vi "main OP300.vi"() -> ()   [LabVIEW 2020]
uses:
  SubVI/OP300ZP_state.ctl
  <vilib>/Sylvain.lib/02 SLIM ZEN WS 500/SubVi/FGV.ctl
  <vilib>/Sylvain.lib/02 SLIM ZEN WS 500/SubVi/VG_progressBar.vi
  SubVI/CheminDeBase.vi
  VG/PN.vi
  VG/IS30%.vi
  VG/R.vi
panel:
  out "IS30% ?":bool
  out "Cluster":T1
  out "VISA OUT":T2
  out "progression":u8(slide) scale=0.0..100.0
  out "PN":string
  out "errout 2":errorcluster={"status"=TRUE, "code"=0, "source"="PCAN_CHANNEL ILLEGAL"} caption="errout"
  out "errout":errorcluster caption="sortie d'erreur"
  out "STOP":bool
  out "TOP":string
  out "DRAW":picture
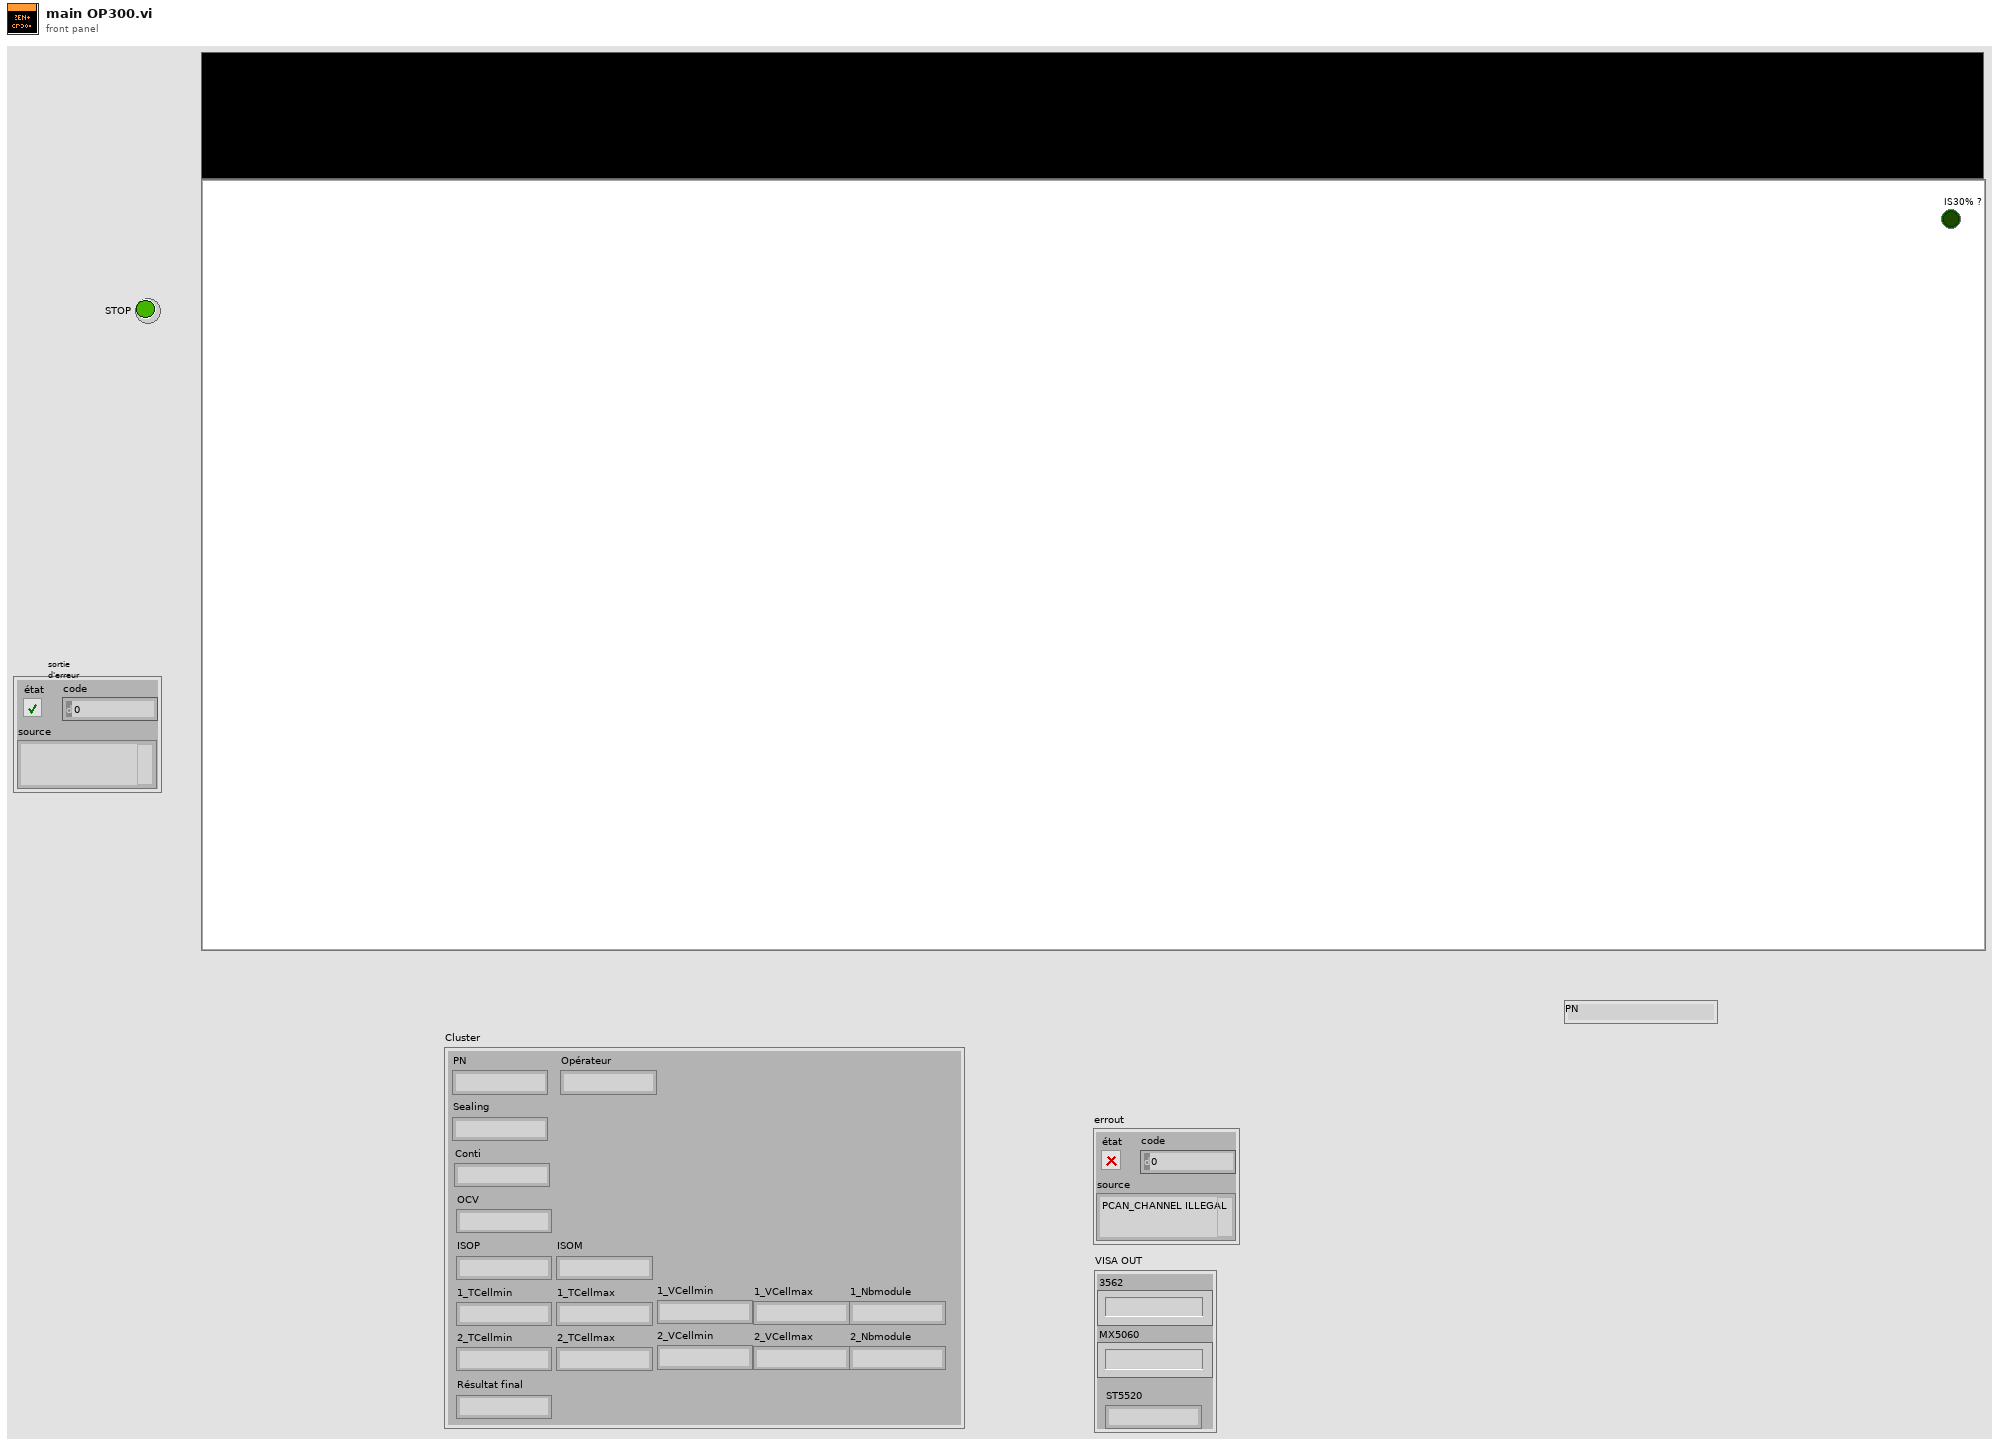
[diagram p1: front panel]
types:
  T1 = cluster{"PN":string, "Opérateur":string, "Sealing":string, "Conti":string, "OCV":string, "ISOP":string, "ISOM":string, "1_TCellmin":string, "1_TCellmax":string, "1_VCellmin":string, "1_VCellmax":string, "1_Nbmodule":string, "2_TCellmin":string, "2_TCellmax":string, "2_VCellmin":string, "2_VCellmax":string, "2_Nbmodule":string, "Résultat final":string}
  T2 = cluster{"3562":string, "MX5060":string, "ST5520":string}
  T3 = cluster{"PN":string, "Sealing":string, "Opérateur":string, "Conti":string, "OCV":string, "ISOP":string, "ISOM":string, "1_TCellmin":string, "1_TCellmax":string, "1_VCellmin":string, "1_VCellmax":string, "1_Nbmodule":string, "2_TCellmin":string, "2_TCellmax":string, "2_VCellmin":string, "2_VCellmax":string, "2_Nbmodule":string, "Résultat final":string}
  T4 = typedef "OP300ZP_state.ctl" = enum16{"Null", "Demarrage", "Init", "Scan", "Montage", "Conti", "OCV", "Iso", "Vpack", "DataDyn", "Dessouter", "DataDyn2", "Demontage", "Crash", "Next", "Sealing", "Comext"}
  T5 = typedef "FGV.ctl" = enum16{"GET", "SET", "RAZ"}
  T6 = cluster{"1_TCellmin":string, "1_TCellmax":string, "1_VCellmin":string, "1_VCellmax":string, "1_Nbmodule":string}
  T7 = cluster{"Chaîne":string, "Chaîne":string, "Chaîne":string, "Chaîne":string, "Chaîne":string, "Chaîne":string, "Chaîne":string, "Chaîne 2":string}
  T8 = typedef "imagedata.ctl" = cluster{"image type":i32, "image depth":i32, "image":u8[], "mask":u8[], "colors":u32[], "Rectangle":cluster{"left":i16, "top":i16, "right":i16, "bottom":i16}}
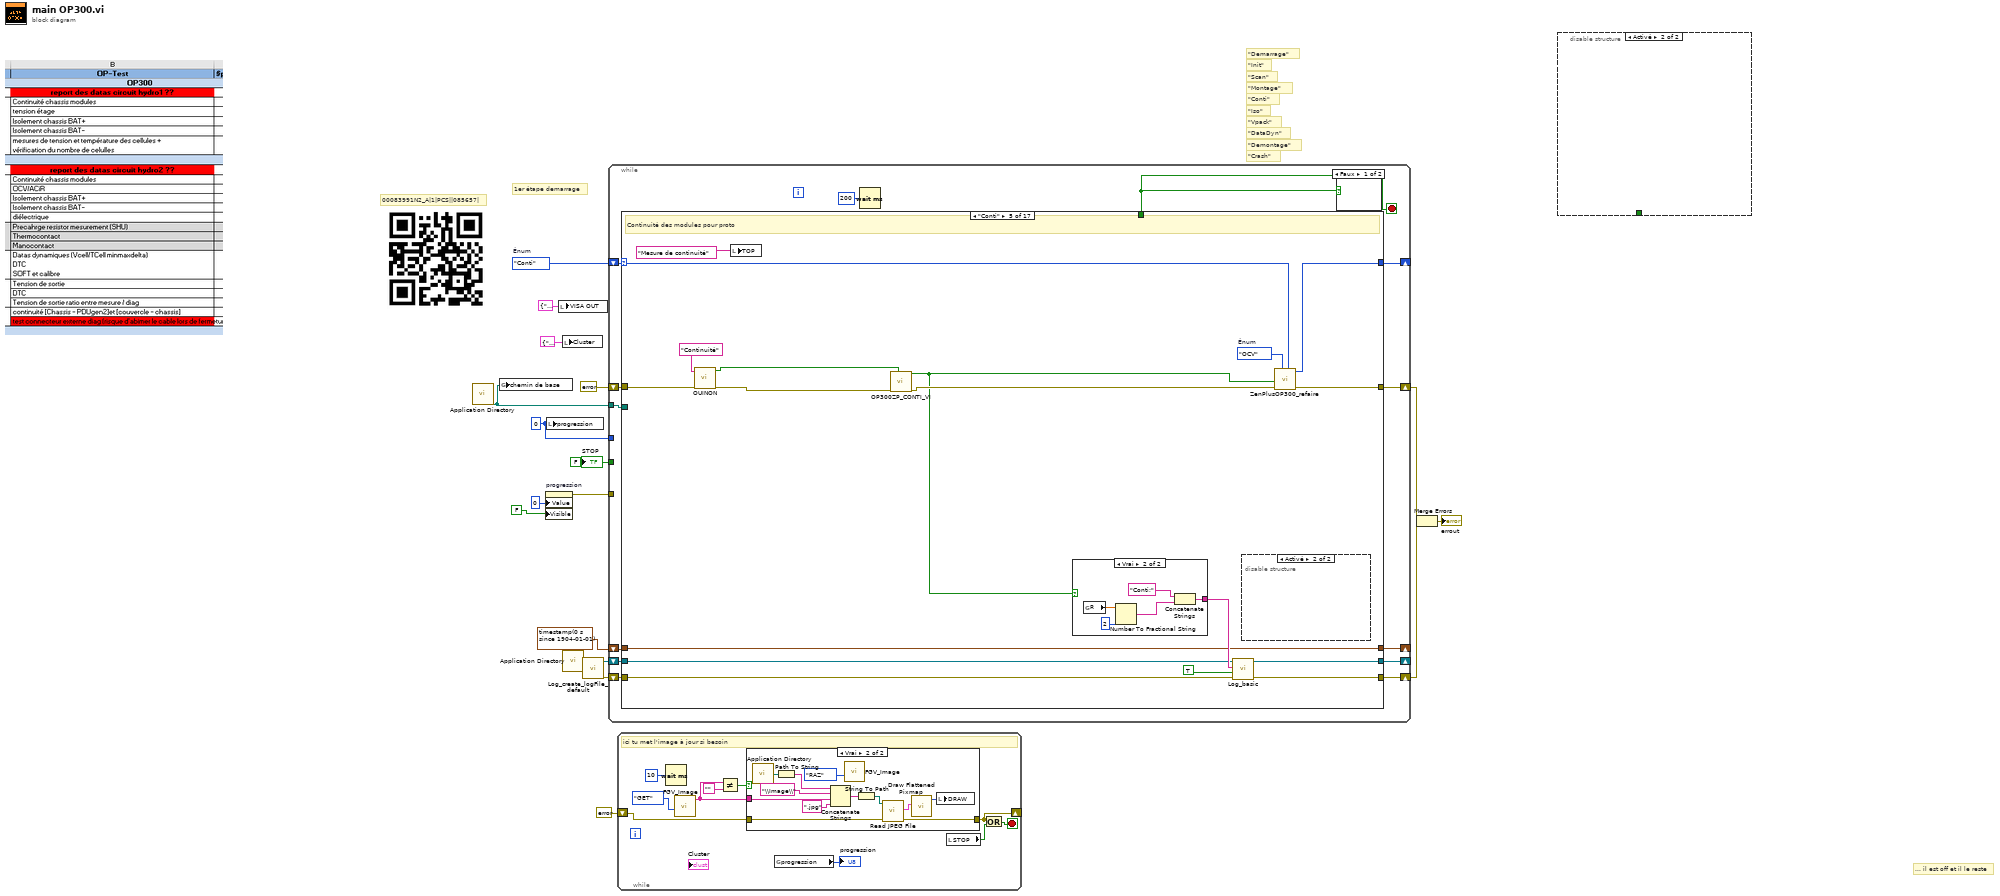
[diagram p0: block diagram]
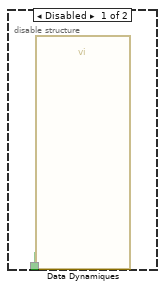
[diagram p2: hidden frame]
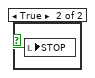
[diagram p4: hidden frame]
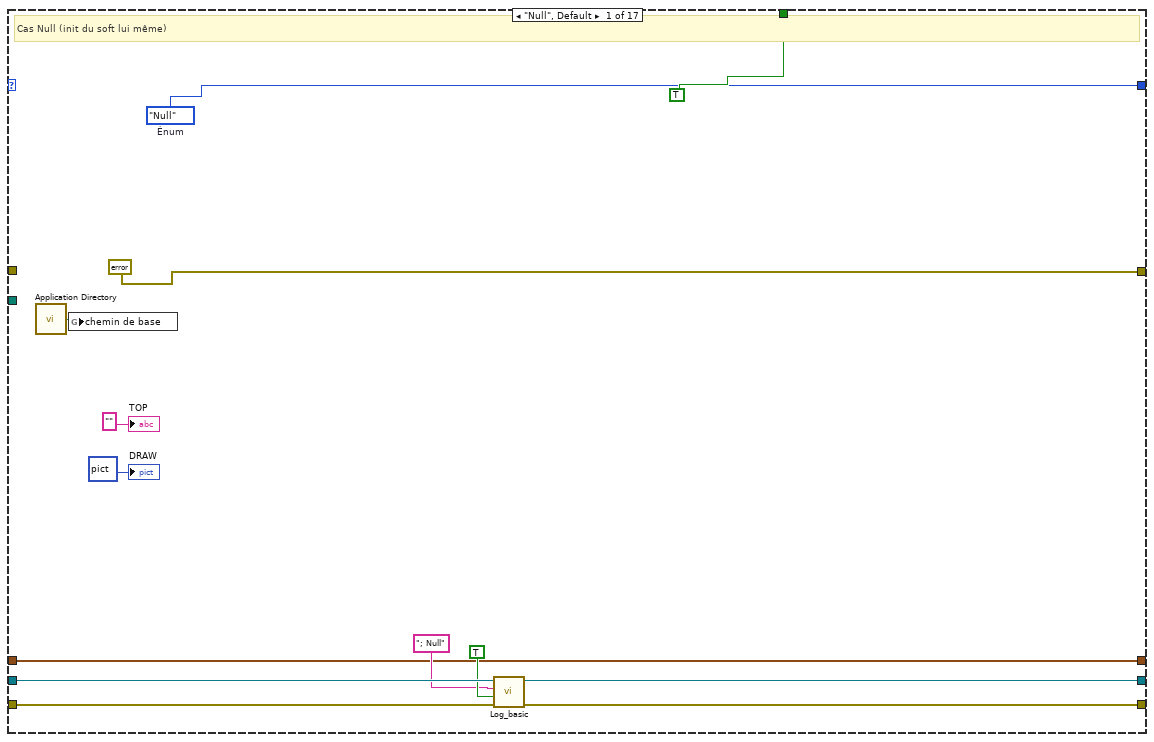
[diagram p5: hidden frame]
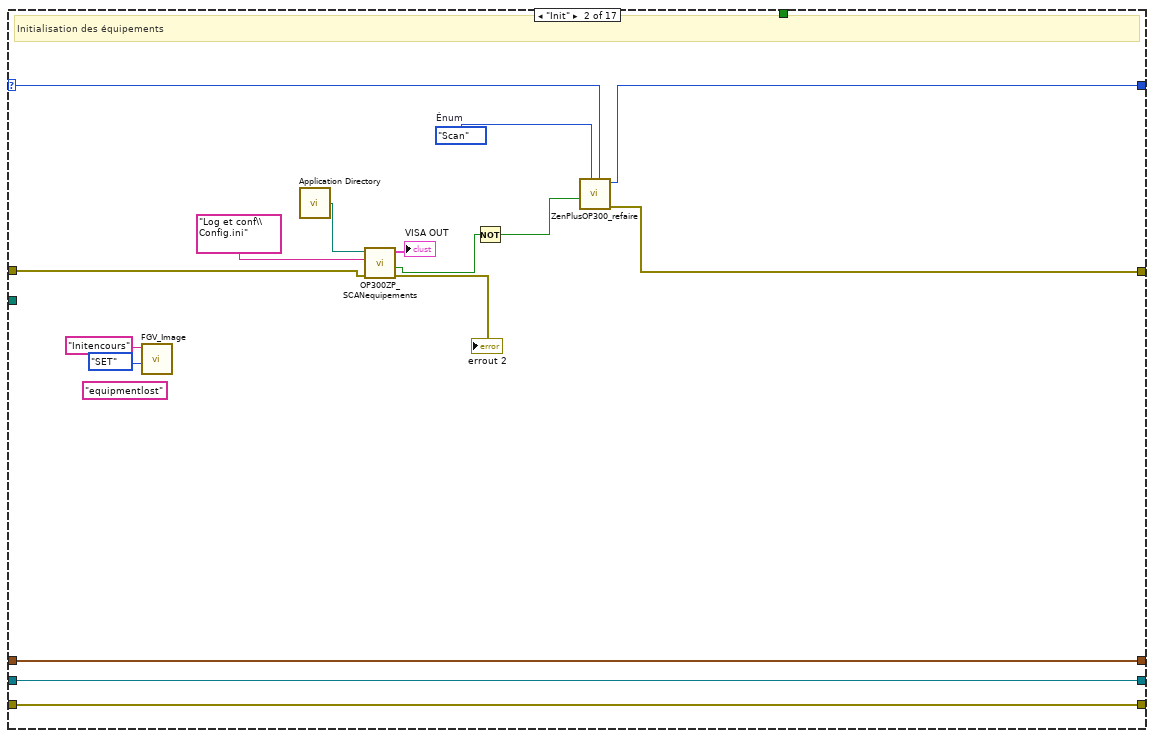
[diagram p6: hidden frame]
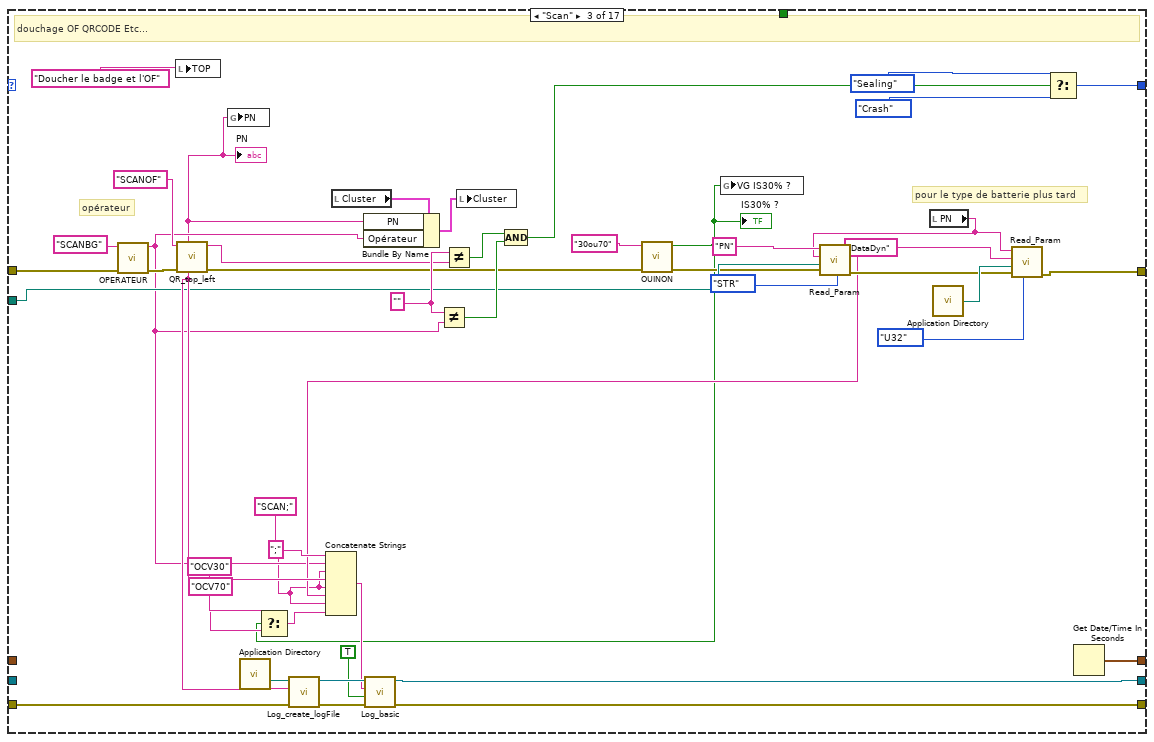
[diagram p7: hidden frame]
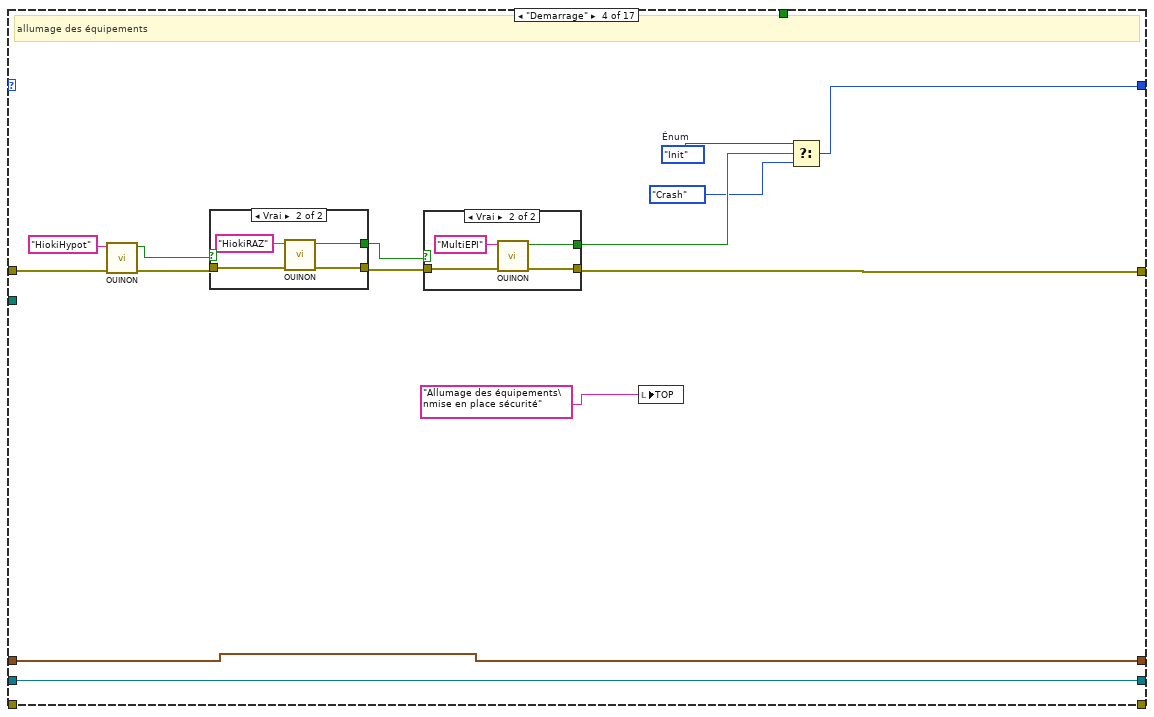
[diagram p8: hidden frame]
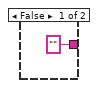
[diagram p11: hidden frame]
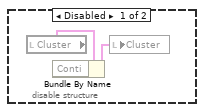
[diagram p12: hidden frame]
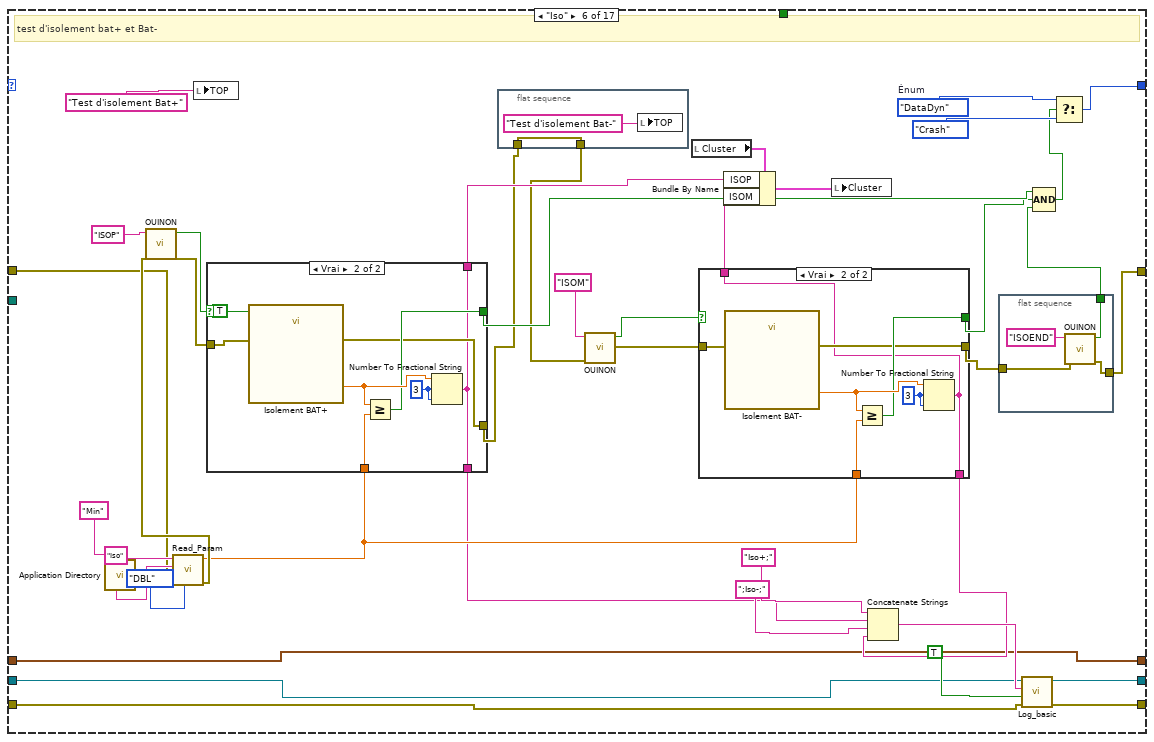
[diagram p13: hidden frame]
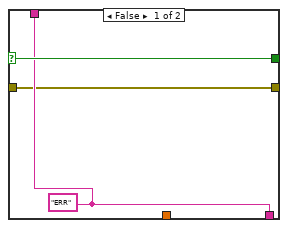
[diagram p14: hidden frame]
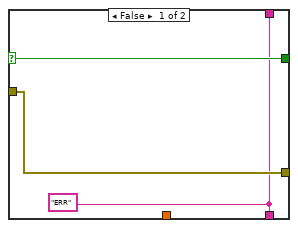
[diagram p15: hidden frame]
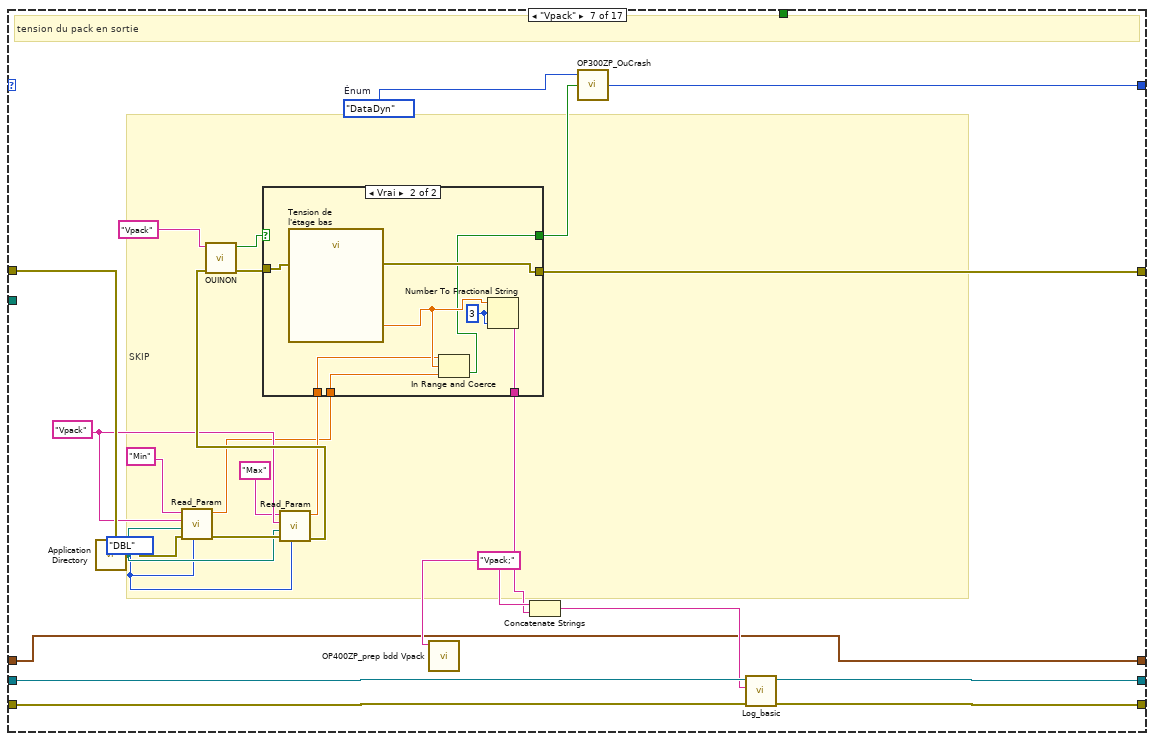
[diagram p16: hidden frame]
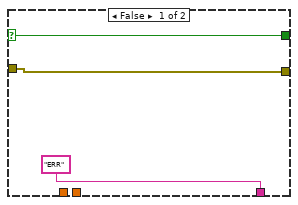
[diagram p17: hidden frame]
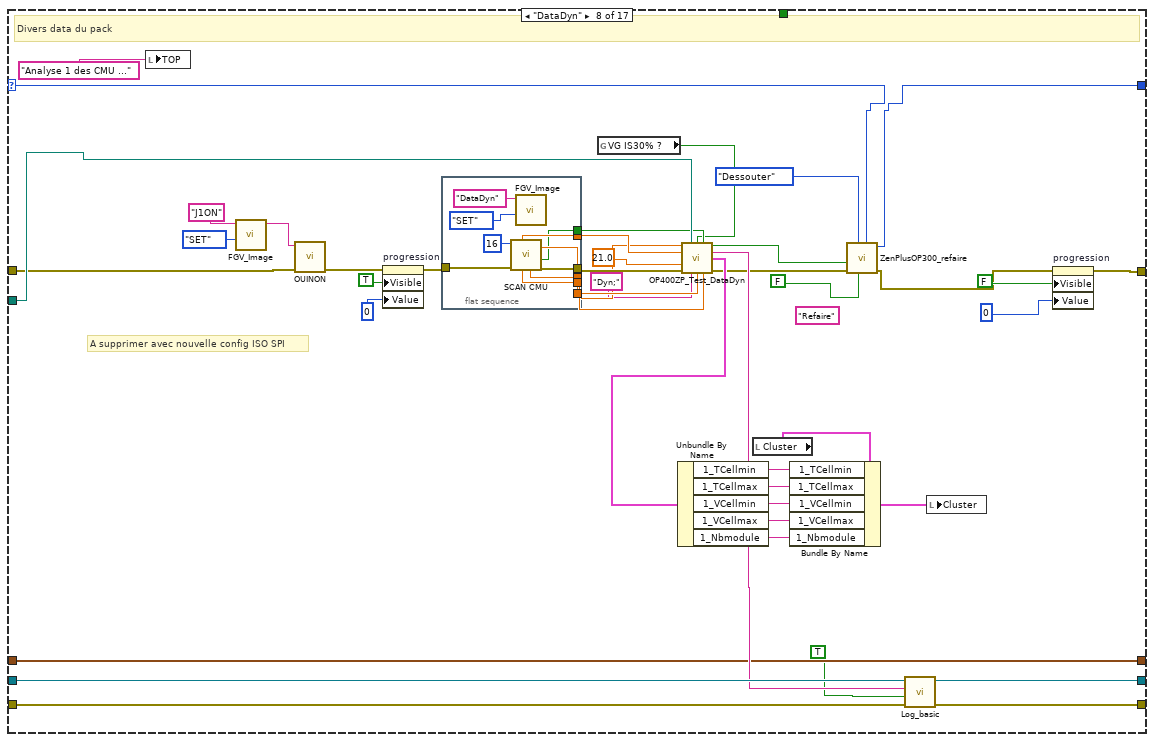
[diagram p18: hidden frame]
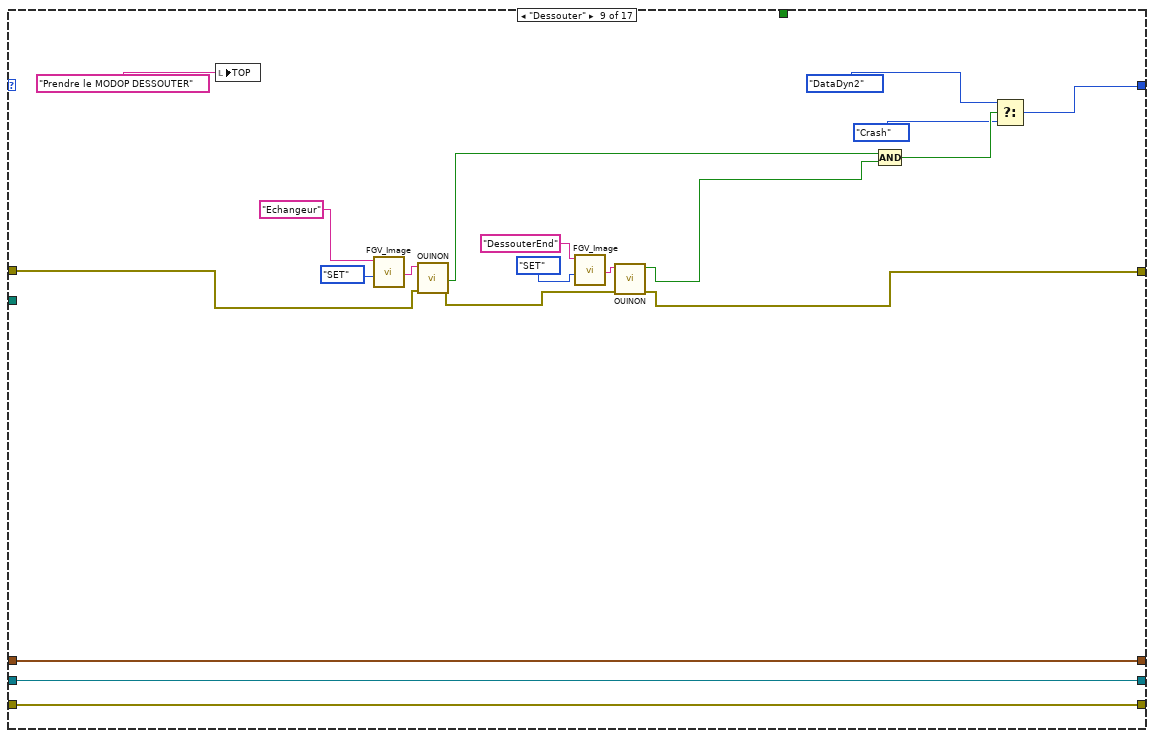
[diagram p19: hidden frame]
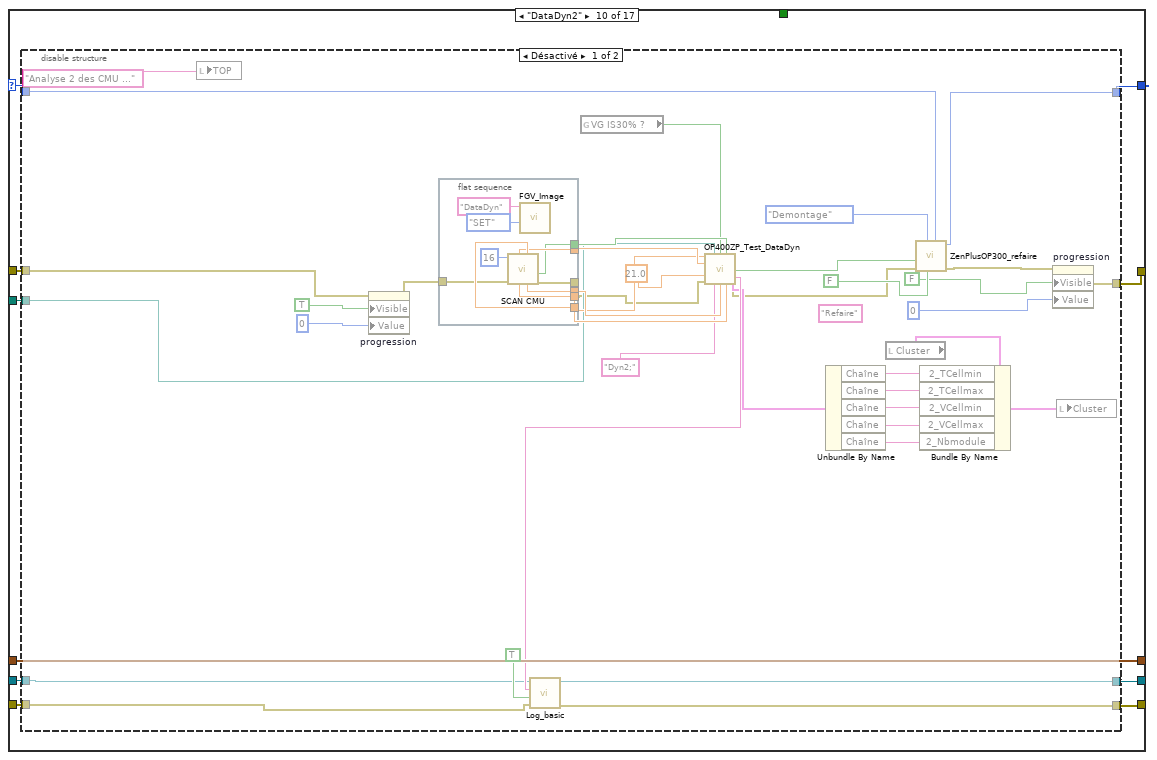
[diagram p20: hidden frame]
diagram:
  w7 = u8 0 ("progression")
  w8 = OP300ZP_state."Conti"  # Énum
  w14 = FALSE ("STOP")
  # "00083991N2_A|1|PCS||085657|"
  # "1er étape demarrage"
  # "\"Crash\""
  # "\"Demontage\""
  # "\"DataDyn\""
  # "\"Iso\""
  # "\"Montage\""
  # "\"Scan\""
  # "\"Init\""
  # "\"Demarrage\""
  # "\"Conti\""
  # "\"Vpack\""
  # "... il est off et il le reste"
  n1 = call <vilib>:"Application Directory.vi"() -> ("Application Directory"=w13:path)
  n2 = global write "CheminDeBase.vi" "chemin de base"(w13) -> ()
  n3 = property on="progression" class="Gliss (strict)"("Value"=u8 0 ("progression"), "Visible"=FALSE) -> (error out=w5:errorcluster)  [unwired: 2 in, 1 out]
  n4 = local write "progression"(w7) -> ()
  n5 = local write "VISA OUT"(T2 {"3562"="", "MX5060"="", "ST5520"=""} ("VISA OUT")) -> ()
  n6 = local write "Cluster"(T3 {"PN"="0", "Sealing"="0", "Opérateur"="0", "Conti"="0", "OCV"="0", "ISOP"="0", "ISOM"="0", "1_TCellmin"="0", "1_TCellmax"="0", "1_VCellmin"="0", "1_VCellmax"="0", "1_Nbmodule"="0", "2_TCellmin"="0", "2_TCellmax"="0", "2_VCellmin"="0", "2_VCellmax"="0", "2_Nbmodule"="0", "Résultat final"="0"} ("Cluster")) -> ()
  n7 = call <vilib>:"Application Directory.vi"() -> ("Application Directory"=w11:path)
  n8 = call <vilib>:"Log_create_logFile_default.vi"("appdir"=w11) -> ("errout"=w12:errorcluster, "Fichier à flux d'octets en sortie"=w15:refnum<file>)  [unwired: 9 in]
  n9 = while {
    shift-right: [w30] -> w17
    shift-left: errorcluster {"status"=FALSE, "code"=0, "source"=""} ("error out") -> [w19]
    shift-right: [w23] -> _
    shift-left: w8 -> [w24]
    shift-right: [w26] -> w16
    shift-left: w12 -> [w29]
    shift-right: [w27] -> _
    shift-left: w15 -> [w28]
    tunnel: w13 -> [w22]
    tunnel: w14 -> [_]
    shift-right: [w20] -> _
    shift-left: timestamp(0 s since 1904-01-01) ("seconds since 1Jan1904") -> [w21]
    tunnel: w7 -> [_]
    tunnel: w5 -> [_]
    stop <- w25 stop-if-true
    n10 = case shown="\"Conti\"" w24 {
      selector: w24 -> [_ w55 _ _ w140 _ _ w299 _ w344 _ _ _ _ _ w533 w585]
      tunnel: w19 -> [_ w58 w107 w120 w138 w160 w241 w297 w320 w336 w404 w413 w438 w457 w493 w529 w606]
      tunnel: [errorcluster {"status"=FALSE, "code"=0, "source"=""} ("errin") w57 w86 w119 w142 w172 w245 w298 w328 w337 w403 w412 w438 w455 w508 w532 w592] -> w30
      tunnel: w29 -> [w41 w61 w103 _ w148 w186 w251 w305 w319 w340 w401 w415 w441 w480 w512 w538 w595]
      tunnel: w28 -> [w42 w60 _ w121 w147 w185 w250 w306 w317 w342 w402 w416 w442 w481 w511 w537 w597]
      tunnel: [w39 w60 w105 w121 w146 w184 w249 w303 w317 w338 w402 w416 _ _ w510 w536 w593] -> w27
      tunnel: [w40 w61 w106 _ w145 w187 w248 w304 w319 w339 w401 w415 w430 w473 w498 w535 w594] -> w26
      tunnel: [TRUE _ _ _ _ _ _ _ _ _ _ FALSE w443 _ _ _ _] -> w25
      tunnel: [w33 w56 w75 w108 w141 w179 w246 w294 w322 w345 w399 w407 OP300ZP_state."Crash" w482 w507 w534 w590] -> w23
      tunnel: w22 -> [_ _ w80 _ _ _ _ w302 _ w343 _ _ _ _ _ w531 _]
      tunnel: w21 -> [w35 w59 _ w118 w144 w180 w228 w300 w318 w341 w400 w411 _ _ w504 w526 w596]
      tunnel: [w35 w59 w94 w118 w144 w180 w228 w300 w318 w341 w400 w411 _ _ w504 w527 w596] -> w20
      frame "Null", Default {
        w33 = OP300ZP_state."Null"  # Énum
        # "Cas Null (init du soft lui même)"
        n11 = call <vilib>:"Application Directory.vi"() -> ("Application Directory"=w45:path)
        n12 = global write "CheminDeBase.vi" "chemin de base"(w45) -> ()
        n13 = call <vilib>:"Log_basic.vi"("errin"=w41, "date?"=TRUE, "chaîne"="; Null", "in"=w42) -> ("sortie d'erreur"=w40:errorcluster, "refnum en sortie"=w39:refnum<file>)  [unwired: 6 in]
        "DRAW" <- picture data[5B] ("DRAW")
        "TOP" <- "" ("TOP")
      }
      frame "Init" {
        w50 = OP300ZP_state."Scan"  # Énum
        (unwired) "equipmentlost" ("image")
        # "Initialisation des équipements"
        n14 = call <vilib>:"FGV_Image.vi"("Énum"=FGV."SET", "IN"="Initencours") -> ()  [unwired: 9 in, 1 out]
        n15 = call <vilib>:"Application Directory.vi"() -> ("Application Directory"=w47:path)
        n16 = call "OP300ZP_SCANequipements.vi"("Errin"=w58, "Chaîne"="Log et conf\\Config.ini", "pathin"=w47) -> ("errout 2"=→"errout 2":errorcluster, "KO?"=w51:bool, "VISA OUT"=→"VISA OUT":T2)  [unwired: 6 in]
        n17 = Not(x=w51) -> (.not. x?=w52:bool)
        n18 = call "ZenPlusOP300_refaire.vi"("refaire"=w55, "casOK"=w50, "test ok ?"=w52) -> ("errout"=w57:errorcluster, "Next"=w56:T4)  [unwired: 7 in]
      }
      frame "Scan" {
        w65 = ";" ("chaîne")
        w97 = "" ("x")
        # "pour le type de batterie plus tard"
        # "opérateur"
        # "douchage OF QRCODE Etc..."
        n19 = call <vilib>:"OPERATEUR.vi"("errin"=w107, "IN"="SCANBG") -> ("error out"=w93:errorcluster, "Dataout"=w71:string)  [unwired: 8 in]
        n20 = local write "TOP"("Doucher le badge et l'OF" ("TOP")) -> ()
        n21 = call <vilib>:"QR_top_left.vi"("errin"=w93, "image"="SCANOF") -> ("error out"=w69:errorcluster, "Réponse"=w91:string, "SN"=w90:string, "PN"=w62:string)  [unwired: 5 in, 1 out]
        "PN" <- w62
        n22 = global write "PN.vi" "PN"(w62) -> ()
        n23 = call <vilib>:"Application Directory.vi"() -> ("Application Directory"=w104:path)
        n24 = call <vilib>:"Log_create_logFile.vi"("errin"=w103, "toute l'expression"=w90, "Application Directory"=w104) -> ("sortie d'erreur"=w101:errorcluster, "Fichier à flux d'octets en sortie"=w102:refnum<file>)  [unwired: 7 in]
        n25 = local read "Cluster"() -> (w73:T1)
        n26 = Bundle By Name(cluster=w73, "PN"=w62, "Opérateur"=w71) -> (w72:T1)
        n27 = Not Equal?(x=w97, y=w71) -> (x != y?=w95:bool)
        n28 = Not Equal?(x=w97, y=w91) -> (x != y?=w96:bool)
        n29 = local write "Cluster"(w72) -> ()
        n30 = Compound Arithmetic op=AND ("Opérateur arithmétique")(w96, w95) -> (w78:bool)
        n31 = call <vilib>:"OUINON.vi"("errin"=w69, "image"="30ou70") -> ("error out"=w68:errorcluster, "OUI/NON"=w63:bool)  [unwired: 8 in]
        "IS30% ?" <- w63
        n32 = Select ("Sélectionner")(t="OCV30" ("section"), s=w63, f="OCV70" ("section")) -> (s? t:f=w64:string)
        n33 = global write "IS30%.vi" "VG IS30% ?"(w63) -> ()
        n34 = local read "PN"() -> (w82:string)
        n35 = call "Read_Param.vi"("Énum"=enum16{"STR", "DBL", "U32"}."STR", "errin"=w68, "pathin"=w80, "section"=w82, "key"="PN") -> ("error out"=w85:errorcluster, "str"=w81:string)  [unwired: 2 in, 3 out]
        n36 = Concatenate Strings("SCAN;" ("chaîne"), w71, w65, w90, w65, w81, w65, w64) -> (w99:string)
        n37 = call <vilib>:"Log_basic.vi"("errin"=w101, "date?"=TRUE, "chaîne"=w99, "in"=w102) -> ("sortie d'erreur"=w106:errorcluster, "refnum en sortie"=w105:refnum<file>)  [unwired: 6 in]
        n38 = call <vilib>:"Application Directory.vi"() -> ("Application Directory"=w89:path)
        n39 = call "Read_Param.vi"("Énum"=enum16{"STR", "DBL", "U32"}."U32", "errin"=w85, "pathin"=w89, "section"="DataDyn", "key"=w82) -> ("error out"=w86:errorcluster)  [unwired: 2 in, 4 out]
        n40 = Select ("Sélectionner")(t=OP300ZP_state."Sealing" ("Énum"), s=w78, f=OP300ZP_state."Crash" ("cas faux")) -> (s? t:f=w75:T4)
        n41 = Get Date/Time In Seconds() -> (seconds since 1Jan1904=w94:timestamp)
      }
      frame "Demarrage" {
        w110 = OP300ZP_state."Init"  # Énum
        # "allumage des équipements"
        n42 = call <vilib>:"OUINON.vi"("errin"=w120, "image"="HiokiHypot") -> ("error out"=w116:errorcluster, "OUI/NON"=w113:bool)  [unwired: 8 in]
        n43 = case shown="Vrai" w113 {
          selector: w113 -> [w123 _]
          tunnel: [w123 w127] -> w114
          tunnel: [w122 w126] -> w115
          tunnel: w116 -> [w122 w124]
          frame False {
          }
          frame True {
            n44 = call <vilib>:"OUINON.vi"("errin"=w124, "image"="HiokiRAZ" ("IN")) -> ("error out"=w126:errorcluster, "OUI/NON"=w127:bool)  [unwired: 8 in]
          }
        }
        n45 = case shown="Vrai" w114 {
          selector: w114 -> [w129 _]
          tunnel: [w129 w133] -> w111
          tunnel: [w128 w132] -> w119
          tunnel: w115 -> [w128 w130]
          frame False {
          }
          frame True {
            n46 = call <vilib>:"OUINON.vi"("errin"=w130, "image"="MultiEPI" ("IN")) -> ("error out"=w132:errorcluster, "OUI/NON"=w133:bool)  [unwired: 8 in]
          }
        }
        n47 = local write "TOP"("Allumage des équipements\nmise en place sécurité" ("TOP")) -> ()
        n48 = Select ("Sélectionner")(t=w110, s=w111, f=OP300ZP_state."Crash" ("cas faux")) -> (s? t:f=w108:T4)
      }
      frame "Conti" {
        w139 = OP300ZP_state."OCV"  # Énum
        # "Continuité des modules pour proto"
        n49 = call <vilib>:"OUINON.vi"("errin"=w138, "image"="Continuité" ("IN")) -> ("error out"=w137:errorcluster, "OUI/NON"=w135:bool)  [unwired: 8 in]
        n50 = local write "TOP"("Mesure de continuité" ("TOP")) -> ()
        n51 = call "OP300ZP_CONTI_VI.vi"("OUI/NON"=w135, "entrée d'erreur (pas d'erreur)"=w137) -> ("sortie d'erreur"=w136:errorcluster, "Dernier Point 3"=w134:bool)  [unwired: 6 in, 2 out]
        n52 = case shown="Vrai" w134 {
          tunnel: ["" w157] -> w150
          frame False {
          }
          frame True {
            n53 = global read "R.vi" "R"() -> (w155:dbl)
            n54 = Number To Fractional String(number=w155, precision (6)=i16 2 ("précision (6)")) -> (F-format string=w154:string)  [unwired: 2 in]
            n55 = Concatenate Strings("Conti;" ("chaîne"), w154) -> (w157:string)
          }
        }
        n56 = call <vilib>:"Log_basic.vi"("errin"=w148, "date?"=TRUE, "chaîne"=w150, "in"=w147) -> ("sortie d'erreur"=w145:errorcluster, "refnum en sortie"=w146:refnum<file>)  [unwired: 6 in]
        n57 = disable-structure shown="Activé" {
          frame Disabled {
            n58 = local read "Cluster"() -> (w159:T1)
            n59 = Bundle By Name(cluster=w159) -> (w158:T1)  [unwired: 1 in]
            n60 = local write "Cluster"(w158) -> ()
          }
          frame Enabled {
          }
        }
        n61 = call "ZenPlusOP300_refaire.vi"("refaire"=w140, "casOK"=w139, "errin"=w136, "test ok ?"=w134) -> ("errout"=w142:errorcluster, "Next"=w141:T4)  [unwired: 6 in]
      }
      frame "Iso" {
        w178 = OP300ZP_state."DataDyn"  # Énum
        # "test d'isolement bat+ et Bat-"
        n62 = call <vilib>:"Application Directory.vi"() -> ("Application Directory"=w195:path)
        n63 = call "Read_Param.vi"("Énum"=enum16{"STR", "DBL", "U32"}."DBL", "errin"=w160, "pathin"=w195, "section"="Iso", "key"="Min") -> ("error out"=w192:errorcluster, "dbl"=w189:dbl)  [unwired: 2 in, 3 out]
        n64 = call <vilib>:"OUINON.vi"("errin"=w192, "image"="ISOP" ("IN")) -> ("error out"=w165:errorcluster, "OUI/NON"=w166:bool)  [unwired: 8 in]
        n65 = local write "TOP"("Test d'isolement Bat+" ("TOP")) -> ()
        n66 = case shown="Vrai" w166 {
          selector: w166 -> [w217 _]
          tunnel: w165 -> [w218 w226]
          tunnel: [w218 w221] -> w163
          tunnel: [w216 w220] -> w182
          tunnel: [w217 w222] -> w170
          tunnel: w189 -> [_ w224]
          tunnel: [w216 w220] -> w174
          frame False {
            w216 = "ERR"
          }
          frame True {
            w225 = i16 3 ("largeur (-)")
            n67 = call "Isolement BAT+"("Enable"=TRUE, "error in (no error)"=w226) -> ("ISOP"=w223:dbl, "error out"=w221:errorcluster)  [unwired: 15 in, 1 out]
            n68 = Greater Or Equal?(x=w223, y=w224) -> (x >= y?=w222:bool)
            n69 = Number To Fractional String(number=w223, width (-)=w225, precision (6)=w225) -> (F-format string=w220:string)  [unwired: 1 in]
          }
        }
        n70 = flat-sequence {
          tunnel: w163 -> [w200]
          tunnel: [w200] -> w162
          frame #0 {
            n71 = local write "TOP"("Test d'isolement Bat-" ("TOP")) -> ()
          }
        }
        n72 = call <vilib>:"OUINON.vi"("errin"=w162, "image"="ISOM" ("IN")) -> ("error out"=w164:errorcluster, "OUI/NON"=w190:bool)  [unwired: 8 in]
        n73 = local read "Cluster"() -> (w176:T1)
        n74 = case shown="Vrai" w190 {
          selector: w190 -> [w208 _]
          tunnel: [w206 w211] -> w171
          tunnel: [w207 w210] -> w181
          tunnel: [w208 w212] -> w169
          tunnel: w189 -> [_ w214]
          tunnel: [w207 w210] -> w173
          tunnel: w164 -> [w206 w209]
          frame False {
            w207 = "ERR"
          }
          frame True {
            w215 = i16 3 ("largeur (-)")
            n75 = call "Isolement BAT-"("error in (no error)"=w209) -> ("ISOM"=w213:dbl, "error out"=w211:errorcluster)  [unwired: 16 in, 1 out]
            n76 = Greater Or Equal?(x=w213, y=w214) -> (x >= y?=w212:bool)
            n77 = Number To Fractional String(number=w213, width (-)=w215, precision (6)=w215) -> (F-format string=w210:string)  [unwired: 1 in]
          }
        }
        n78 = Bundle By Name(cluster=w176, "ISOP"=w174, "ISOM"=w173) -> (w175:T1)
        n79 = local write "Cluster"(w175) -> ()
        n80 = Concatenate Strings("Iso+;" ("chaîne"), w182, ";Iso-;" ("chaîne"), w181) -> (w198:string)
        n81 = flat-sequence {
          tunnel: [w203] -> w172
          tunnel: w171 -> [w204]
          tunnel: [w202] -> w168
          frame #0 {
            n82 = call <vilib>:"OUINON.vi"("errin"=w204, "image"="ISOEND") -> ("error out"=w203:errorcluster, "OUI/NON"=w202:bool)  [unwired: 8 in]
          }
        }
        n83 = call <vilib>:"Log_basic.vi"("errin"=w186, "date?"=TRUE, "chaîne"=w198, "in"=w185) -> ("sortie d'erreur"=w187:errorcluster, "refnum en sortie"=w184:refnum<file>)  [unwired: 6 in]
        n84 = Compound Arithmetic op=AND ("Opérateur arithmétique")(w170, w169, w168) -> (w167:bool)
        n85 = Select ("Sélectionner")(t=w178, s=w167, f=OP300ZP_state."Crash" ("cas faux")) -> (s? t:f=w179:T4)
      }
      frame "Vpack" {
        w227 = OP300ZP_state."DataDyn"  # Énum
        w236 = enum16{"STR", "DBL", "U32"}."DBL" ("Énum")
        w239 = "Vpack" ("section")
        # "SKIP"
        # "tension du pack en sortie"
        n86 = call <vilib>:"Application Directory.vi"() -> ("Application Directory"=w237:path)
        n87 = call "Read_Param.vi"("Énum"=w236, "errin"=w241, "pathin"=w237, "section"=w239, "key"="Min") -> ("error out"=w242:errorcluster, "dbl"=w234:dbl)  [unwired: 2 in, 3 out]
        n88 = call "Read_Param.vi"("Énum"=w236, "errin"=w242, "pathin"=w237, "section"=w239, "key"="Max") -> ("error out"=w240:errorcluster, "dbl"=w235:dbl)  [unwired: 2 in, 3 out]
        n89 = call <vilib>:"OUINON.vi"("errin"=w240, "image"="Vpack" ("IN")) -> ("error out"=w244:errorcluster, "OUI/NON"=w231:bool)  [unwired: 8 in]
        n90 = case shown="Vrai" w231 {
          selector: w231 -> [w252 _]
          tunnel: w244 -> [w254 w262]
          tunnel: [w254 w259] -> w245
          tunnel: ["ERR" w260] -> w229
          tunnel: [w252 w257] -> w230
          tunnel: w235 -> [_ w255]
          tunnel: w234 -> [_ w256]
          frame False {
          }
          frame True {
            w261 = i16 3 ("largeur (-)")
            n91 = call "Tension de l'étage bas"("error in (no error)"=w262) -> ("Vpack"=w258:dbl, "error out"=w259:errorcluster)  [unwired: 16 in, 1 out]
            n92 = In Range and Coerce(upper limit=w255, x=w258, lower limit=w256) -> (In Range?=w257:bool)  [unwired: 1 out]
            n93 = Number To Fractional String(number=w258, width (-)=w261, precision (6)=w261) -> (F-format string=w260:string)  [unwired: 1 in]
          }
        }
        n94 = call "OP400ZP_prep bdd Vpack.vi"("OCV"=w229) -> ()  [unwired: 10 in, 1 out]
        n95 = Concatenate Strings("Vpack;" ("chaîne"), w229) -> (w232:string)
        n96 = call "OP300ZP_OuCrash.vi"("Booléen"=w230, "in"=w227) -> ("OUT"=w246:T4)  [unwired: 1 in]
        n97 = call <vilib>:"Log_basic.vi"("errin"=w251, "chaîne"=w232, "in"=w250) -> ("sortie d'erreur"=w248:errorcluster, "refnum en sortie"=w249:refnum<file>)  [unwired: 7 in]
      }
      frame "DataDyn" {
        (unwired) "Refaire" ("image")
        # "A supprimer avec nouvelle config ISO SPI"
        # "Divers data du pack"
        n98 = local write "TOP"("Analyse 1 des CMU ..." ("TOP")) -> ()
        n99 = call <vilib>:"FGV_Image.vi"("Énum"=FGV."SET", "IN"="J1ON") -> ("OUT"=w278:string)  [unwired: 9 in]
        n100 = call <vilib>:"OUINON.vi"("errin"=w297, "image"=w278) -> ("error out"=w277:errorcluster)  [unwired: 8 in, 1 out]
        n101 = property on="progression" class="Gliss (strict)"(error in=w277, "Visible"=TRUE, "Value"=u8 0 ("progression")) -> (error out=w284:errorcluster)  [unwired: 1 in, 1 out]
        n102 = flat-sequence {
          tunnel: [w316] -> w293
          tunnel: [w315] -> w292
          tunnel: [w314] -> w291
          tunnel: [w313] -> w290
          tunnel: [w312] -> w289
          tunnel: [w311] -> w288
          tunnel: w284 -> [w310]
          frame #0 {
            n103 = call "SCAN CMU.vi"("errin"=w310, "Nb modules"=i16 16) -> ("errout"=w316:errorcluster, "# température + #tension OK?"=w311:bool, "Vmin"=w315:dbl, "Vmax"=w314:dbl, "Tmin"=w312:dbl, "Tmax"=w313:dbl)  [unwired: 4 out]
            n104 = call <vilib>:"FGV_Image.vi"("Énum"=FGV."SET", "IN"="DataDyn") -> ()  [unwired: 9 in, 1 out]
          }
        }
        n105 = global read "IS30%.vi" "VG IS30% ?"() -> (w263:bool)
        n106 = call "OP400ZP_Test_DataDyn.vi"("Tcell Min (°C)"=w289, "appdir"=w302, "is30%?"=w263, "MCU"=w288, "Tcell Max (°C)"=w290, "Température usine (°C)"=21.0, "errin"=w293, "testname"="Dyn;", "Vcell Min (V)"=w292, "Vcell Max (V)"=w291) -> ("pass"=w264:bool, "datalog"=w301:string, "Cluster"=w272:T6, "errout"=w265:errorcluster)  [unwired: 1 in, 1 out]
        n107 = Unbundle By Name(w272) -> ("1_TCellmin"=w271:string, "1_TCellmax"=w270:string, "1_VCellmin"=w269:string, "1_VCellmax"=w268:string, "1_Nbmodule"=w267:string)
        n108 = local read "Cluster"() -> (w274:T1)
        n109 = Bundle By Name(cluster=w274, "1_TCellmin"=w271, "1_TCellmax"=w270, "1_VCellmin"=w269, "1_VCellmax"=w268, "1_Nbmodule"=w267) -> (w273:T1)
        n110 = call "ZenPlusOP300_refaire.vi"("refaire"=w299, "Pédale"=FALSE, "casOK"=OP300ZP_state."Dessouter" ("Énum"), "errin"=w265, "test ok ?"=w264) -> ("errout"=w266:errorcluster, "Next"=w294:T4)  [unwired: 5 in]
        n111 = call <vilib>:"Log_basic.vi"("errin"=w305, "date?"=TRUE, "chaîne"=w301, "in"=w306) -> ("sortie d'erreur"=w304:errorcluster, "refnum en sortie"=w303:refnum<file>)  [unwired: 6 in]
        n112 = local write "Cluster"(w273) -> ()
        n113 = property on="progression" class="Gliss (strict)"(error in=w266, "Visible"=FALSE, "Value"=u8 0 ("progression")) -> (error out=w298:errorcluster)  [unwired: 1 in, 1 out]
      }
      frame "Dessouter" {
        n114 = local write "TOP"("Prendre le MODOP DESSOUTER" ("TOP")) -> ()
        n115 = call <vilib>:"FGV_Image.vi"("Énum"=FGV."SET", "IN"="Echangeur") -> ("OUT"=w333:string)  [unwired: 9 in]
        n116 = call <vilib>:"OUINON.vi"("errin"=w320, "image"=w333) -> ("error out"=w329:errorcluster, "OUI/NON"=w326:bool)  [unwired: 8 in]
        n117 = call <vilib>:"FGV_Image.vi"("Énum"=FGV."SET", "IN"="DessouterEnd") -> ("OUT"=w332:string)  [unwired: 9 in]
        n118 = call <vilib>:"OUINON.vi"("errin"=w329, "image"=w332) -> ("error out"=w328:errorcluster, "OUI/NON"=w327:bool)  [unwired: 8 in]
        n119 = Compound Arithmetic op=AND(w326, w327) -> (w325:bool)
        n120 = Select(t=OP300ZP_state."DataDyn2" ("Next"), s=w325, f=OP300ZP_state."Crash" ("cas faux")) -> (s? t:f=w322:T4)
      }
      frame "DataDyn2" {
        n121 = disable-structure shown="Désactivé" {
          disable-tunnel: [w368 _] -> w345
          disable-tunnel: w344 -> [w367 _]
          disable-tunnel: w343 -> [w366 _]
          disable-tunnel: w342 -> [w365 _]
          disable-tunnel: w340 -> [w364 _]
          disable-tunnel: [w363 _] -> w339
          disable-tunnel: [w362 _] -> w338
          disable-tunnel: [w361 _] -> w337
          disable-tunnel: w336 -> [w350 _]
          frame Disabled {
            (unwired) "Refaire" ("image")
            n122 = local write "TOP"("Analyse 2 des CMU ..." ("TOP")) -> ()
            n123 = property on="progression" class="Gliss (strict)"(error in=w350, "Visible"=TRUE, "Value"=u8 0 ("progression")) -> (error out=w374:errorcluster)  [unwired: 1 in, 1 out]
            n124 = flat-sequence {
              tunnel: [w394] -> w348
              tunnel: [w393] -> w382
              tunnel: [w392] -> w381
              tunnel: [w391] -> w380
              tunnel: [w390] -> w379
              tunnel: [w389] -> w378
              tunnel: w374 -> [w388]
              frame #0 {
                n125 = call "SCAN CMU.vi"("errin"=w388, "Nb modules"=i16 16) -> ("errout"=w394:errorcluster, "# température + #tension OK?"=w389:bool, "Vmin"=w393:dbl, "Vmax"=w392:dbl, "Tmin"=w390:dbl, "Tmax"=w391:dbl)  [unwired: 4 out]
                n126 = call <vilib>:"FGV_Image.vi"("Énum"=FGV."SET", "IN"="DataDyn") -> ()  [unwired: 9 in, 1 out]
              }
            }
            n127 = global read "IS30%.vi" "VG IS30% ?"() -> (w346:bool)
            n128 = call "OP400ZP_Test_DataDyn.vi"("Tcell Min (°C)"=w379, "appdir"=w366, "is30%?"=w346, "MCU"=w378, "Tcell Max (°C)"=w380, "Température usine (°C)"=21.0, "errin"=w348, "testname"="Dyn2;", "Vcell Min (V)"=w382, "Vcell Max (V)"=w381) -> ("pass"=w347:bool, "datalog"=w384:string, "StrData"=w352:T7, "errout"=w349:errorcluster)  [unwired: 1 in, 1 out]
            n129 = call <vilib>:"Log_basic.vi"("errin"=w364, "date?"=TRUE, "chaîne"=w384, "in"=w365) -> ("sortie d'erreur"=w363:errorcluster, "refnum en sortie"=w362:refnum<file>)  [unwired: 6 in]
            n130 = Unbundle By Name(w352) -> ("Chaîne"=w357:string, "Chaîne"=w356:string, "Chaîne"=w355:string, "Chaîne"=w354:string, "Chaîne"=w353:string)
            n131 = local read "Cluster"() -> (w359:T1)
            n132 = call "ZenPlusOP300_refaire.vi"("refaire"=w367, "Pédale"=FALSE, "casOK"=OP300ZP_state."Demontage" ("Énum"), "errin"=w349, "test ok ?"=w347) -> ("errout"=w370:errorcluster, "Next"=w368:T4)  [unwired: 5 in]
            n133 = Bundle By Name(cluster=w359, "2_TCellmin"=w357, "2_TCellmax"=w356, "2_VCellmin"=w355, "2_VCellmax"=w354, "2_Nbmodule"=w353) -> (w358:T1)
            n134 = property on="progression" class="Gliss (strict)"(error in=w370, "Visible"=FALSE, "Value"=u8 0 ("progression")) -> (error out=w361:errorcluster)  [unwired: 1 in, 1 out]
            n135 = local write "Cluster"(w358) -> ()
          }
          frame Enabled {
          }
        }
      }
      frame "Montage" {
        w397 = OP300ZP_state."Conti"  # Énum
        # "montage du produit sur le banc"
        n136 = local write "TOP"("Montage du pack" ("TOP")) -> ()
        n137 = call <vilib>:"OUINON.vi"("errin"=w404, "image"="Montage" ("IN")) -> ("error out"=w403:errorcluster, "OUI/NON"=w398:bool)  [unwired: 8 in]
        n138 = Select ("Sélectionner")(t=w397, s=w398, f=OP300ZP_state."Crash" ("cas faux")) -> (s? t:f=w399:T4)
      }
      frame "Demontage" {
        w409 = OP300ZP_state."Next"  # Énum
        n139 = call <vilib>:"OUINON.vi"("errin"=w413, "image"="Demontage" ("IN")) -> ("error out"=w412:errorcluster, "OUI/NON"=w410:bool)  [unwired: 8 in]
        n140 = Select ("Sélectionner")(t=w409, s=w410, f=OP300ZP_state."Crash" ("cas faux")) -> (s? t:f=w407:T4)
        n141 = local write "TOP"("Demontage du pack" ("TOP")) -> ()
      }
      frame "Crash" {
        # "\\\\forseepower.com\\fr\\040 Production\\FR7 - Poitiers\\06 Production\\05. Electronique\\Documents Control lib\\Archives\\ZEN PLUS"
        n142 = Close File(refnum=w442, error in=w441) -> (path=w428:path, error out=w433:errorcluster)
        n143 = call <vilib>:"waitXms.vi"("attente (ms)"=u32 300, "errin"=w433) -> ("errout"=w429:errorcluster)  [unwired: 13 in]
        n144 = local read "Cluster"() -> (w422:T1)
        n145 = Read from Text File(file (use dialog)=w428, error in=w429) -> (text=w427:string, error out=w425:errorcluster)  [unwired: 2 in, 2 out]
        n146 = call "OP300ZP_SN_Reader.vi"("Fichier txt"=w427) -> ("SN"=w420:string)  [unwired: 10 in]
        n147 = Unbundle By Name(w422) -> ("PN"=w419:string)
        n148 = call <vilib>:"FGV_Image.vi"("Énum"=FGV."SET", "IN"="TeamLeader") -> ()  [unwired: 9 in, 1 out]
        n149 = Concatenate Strings(w419, "-SN" ("chaîne"), w420) -> (w421:string)
        n150 = call "OP300ZP_NouveauDossier.vi"("entrée d'erreur (pas d'erreur)"=w425, "Nom du repertoire (PN SN)"=w421, "Network before adding a new folder"=path "\\\\forseepower.com\\fr/040 Production/FR7 - Poitiers/06 Production/05. Electronique/Documents Control lib/Archives/ZEN PLUS" ("chemin de la cible (utiliser une boîte de dialogue)")) -> ("sortie d'erreur"=w426:errorcluster, "Network after adding a new folder"=w423:path)  [unwired: 7 in]
        n151 = Copy ("Copier")(8:w426, 10:w423, 11:w428) -> (0:w432:errorcluster)  [unwired: 2 in, 2 out]
        n152 = call "PvgeneratorOP300.vi"("errin"=w432, "network"=w423, "path in"=w428) -> ("sortie d'erreur"=w436:errorcluster, "network out"=w435:path)  [unwired: 5 in, 2 out]
        n153 = call <vilib>:"POP_GOOGLE.vi"("error in"=w436, "chemin"=w435) -> ("error out"=w431:errorcluster)  [unwired: 8 in, 1 out]
        n154 = flat-sequence {
          tunnel: [TRUE] -> w443
          tunnel: w430 -> [_]
          frame #0 {
          }
        }
        n155 = disable-structure shown="Désactivé" {
          disable-tunnel: w431 -> [w447 _]
          disable-tunnel: [w444 _] -> w430
          frame Disabled {
            n156 = Select ("Sélectionner")(t="1", s=FALSE ("sélecteur"), f="0" ("cas faux")) -> (s? t:f=w448:string)
            n157 = local read "Cluster"() -> (w451:T1)
            n158 = Bundle By Name(cluster=w451, "Résultat final"=w448) -> (w446:T1)
            n159 = call "BDD_2.vi"("errin"=w447, "Cluster"=w446) -> ("error out"=w444:errorcluster)  [unwired: 8 in, 1 out]
          }
          frame Enabled {
          }
        }
      }
      frame "Next" {
        w478 = OP300ZP_state."Null"  # Énum
        w479 = OP300ZP_state."Scan"  # Énum
        # "\\\\forseepower.com\\fr\\040 Production\\FR7 - Poitiers\\06 Production\\05. Electronique\\Documents Control lib\\Archives\\ZEN PLUS"
        n160 = Close File(refnum=w481, error in=w480) -> (path=w458:path, error out=w477:errorcluster)
        n161 = call <vilib>:"waitXms.vi"("attente (ms)"=u32 300, "errin"=w477) -> ("errout"=w470:errorcluster)  [unwired: 13 in]
        n162 = local read "Cluster"() -> (w463:T1)
        n163 = Read from Text File(file (use dialog)=w458, error in=w470) -> (text=w468:string, error out=w467:errorcluster)  [unwired: 2 in, 2 out]
        n164 = call "OP300ZP_SN_Reader.vi"("Fichier txt"=w468) -> ("SN"=w460:string)  [unwired: 10 in]
        n165 = Unbundle By Name(w463) -> ("PN"=w462:string)
        n166 = Concatenate Strings(w462, "-SN" ("chaîne"), w460) -> (w459:string)
        n167 = call "Multi_OUI_NON.vi"("errin"=w457, "errinb"=TRUE, "Tableau"=string[] ["SECU", "Next"]) -> ("errout"=w455:errorcluster, "isok?"=w454:bool)  [unwired: 7 in]
        n168 = call "OP300ZP_NouveauDossier.vi"("entrée d'erreur (pas d'erreur)"=w467, "Nom du repertoire (PN SN)"=w459, "Network before adding a new folder"=path "\\\\forseepower.com\\fr/040 Production/FR7 - Poitiers/06 Production/05. Electronique/Documents Control lib/Archives/ZEN PLUS" ("chemin de la cible (utiliser une boîte de dialogue)")) -> ("sortie d'erreur"=w466:errorcluster, "Network after adding a new folder"=w464:path)  [unwired: 7 in]
        n169 = Copy ("Copier")(8:w466, 10:w464, 11:w458) -> (0:w469:errorcluster)  [unwired: 2 in, 2 out]
        n170 = call "PvgeneratorOP300.vi"("errin"=w469, "network"=w464, "path in"=w458) -> ("sortie d'erreur"=w475:errorcluster, "network out"=w474:path, "tout bon"=w471:bool)  [unwired: 5 in, 1 out]
        n171 = call <vilib>:"POP_GOOGLE.vi"("error in"=w475, "chemin"=w474) -> ("error out"=w472:errorcluster)  [unwired: 8 in, 1 out]
        n172 = Select(t=w479, s=w454, f=w478) -> (s? t:f=w482:T4)
        n173 = disable-structure shown="Désactivé" {
          disable-tunnel: [w490 _] -> w473
          disable-tunnel: w472 -> [w489 _]
          disable-tunnel: w471 -> [w488 _]
          frame Disabled {
            n174 = Select ("Sélectionner")(t="1", s=w488, f="0" ("cas faux")) -> (s? t:f=w484:string)
            n175 = local read "Cluster"() -> (w487:T1)
            n176 = Bundle By Name(cluster=w487, "Résultat final"=w484) -> (w483:T1)
            n177 = call "BDD_2.vi"("errin"=w489, "Cluster"=w483) -> ("error out"=w490:errorcluster)  [unwired: 8 in, 1 out]
          }
          frame Enabled {
          }
        }
      }
      frame "Sealing" {
        w506 = OP300ZP_state."Montage" ("Cas OK")
        # "<30>:(DT):6 Pa"
        # "<20>:(AL):PRESSION HAUTE\n<30>:(DR):-126 Pa\n<30>:(DT):2 Pa\n<30>:(DR):-10 Pa\n<30>:(PB):1 Pa\n<30>:(PB):1 Pa\n<30>:(PB):-2 Pa\n<30>:(DR):-197 Pa\n^C"
        # "SEALING + CONTI BLOC HYDRAU"
        n178 = call <vilib>:"FGV_Image.vi"("Énum"=FGV."SET", "IN"="Sealing") -> ()  [unwired: 9 in, 1 out]
        n179 = call <vilib>:"OUINON.vi"("errin"=w493, "image"="CONTI_HYDRAU") -> ("error out"=w492:errorcluster)  [unwired: 8 in, 1 out]
        n180 = local write "TOP"("Valeur de pression" ("TOP")) -> ()
        n181 = call "OP300ZP_ATEQ.vi"("entrée d'erreur (pas d'erreur)"=w492) -> ("sortie d'erreur"=w496:errorcluster, "Valeur d'étanchéité"=w495:dbl, "Case à cocher"=w494:bool)  [unwired: 8 in]
        n182 = call "ZenPlusOP300_refaire.vi"("refaire"=OP300ZP_state."Sealing", "casOK"=w506, "errin"=w496, "test ok ?"=w494) -> ("errout"=w508:errorcluster, "Next"=w507:T4)  [unwired: 6 in]
        n183 = Equal?(x=w507, y=w506) -> (x = y?=w505:bool)
        n184 = case shown="Vrai" w505 {
          tunnel: w512 -> [w513 w521]
          tunnel: w511 -> [w515 w520]
          tunnel: [w515 w519] -> w510
          tunnel: ["0" w518] -> w499
          tunnel: [w513 w517] -> w498
          tunnel: w495 -> [_ w516]
          frame False {
          }
          frame True {
            n185 = Number To Decimal String(number=w516) -> (decimal integer string=w518:string)  [unwired: 1 in]
            n186 = Concatenate Strings("Sealing;" ("chaîne"), w518) -> (w523:string)
            n187 = call <vilib>:"Log_basic.vi"("errin"=w521, "date?"=TRUE, "chaîne"=w523, "in"=w520) -> ("sortie d'erreur"=w517:errorcluster, "refnum en sortie"=w519:refnum<file>)  [unwired: 6 in]
          }
        }
        n188 = local read "Cluster"() -> (w501:T1)
        n189 = Bundle By Name(cluster=w501, "Sealing"=w499) -> (w500:T1)
        n190 = local write "Cluster"(w500) -> ()
      }
      frame "Comext" {
        n191 = call <vilib>:"OUINON.vi"("errin"=w529, "image"="Comext" ("IN")) -> ("error out"=w528:errorcluster, "OUI/NON"=w525:bool)  [unwired: 8 in]
        n192 = case shown="Vrai" w525 {
          tunnel: w538 -> [w543 w555]
          tunnel: w537 -> [w542 w554]
          tunnel: [w542 w553] -> w536
          tunnel: [w543 w552] -> w535
          tunnel: [OP300ZP_state."Crash" ("OUT") w551] -> w534
          tunnel: w533 -> [_ w550]
          tunnel: [w540 w549] -> w532
          tunnel: w531 -> [_ w548]
          tunnel: w528 -> [w540 w547]
          tunnel: [w541 w546] -> w527
          tunnel: w526 -> [w541 w546]
          frame False {
          }
          frame True {
            (unwired) "Comext;" ("testname")
            w569 = OP300ZP_state."Demontage"  # Énum
            (unwired) "Refaire" ("image")
            n193 = local read "PN"() -> (w566:string)
            n194 = call <vilib>:"Application Directory.vi"() -> ("Application Directory"=w568:path)
            n195 = call "Read_Param.vi"("Énum"=enum16{"STR", "DBL", "U32"}."U32", "errin"=w547, "pathin"=w568, "section"="DataDyn", "key"=w566) -> ("error out"=w561:errorcluster, "U32"=w564:u32)  [unwired: 2 in, 3 out]
            n196 = property on="progression" class="Gliss (strict)"(error in=w561, "Visible"=TRUE, "Value"=u8 0 ("progression")) -> (error out=w560:errorcluster)  [unwired: 1 in, 1 out]
            n197 = call <vilib>:"FGV_Image.vi"("Énum"=FGV."SET", "IN"="DataDyn") -> ()  [unwired: 9 in, 1 out]
            n198 = call "SCAN CMU.vi"("errin"=w560, "Nb modules"=w564) -> ("errout"=w578:errorcluster, "# température + #tension OK?"=w573:bool, "Vmin"=w577:dbl, "Vmax"=w576:dbl, "Tmin"=w574:dbl, "Tmax"=w575:dbl)  [unwired: 4 out]
            n199 = call "OP300ZP_Test_DataDyn.vi"("Vcell Max (V)"=w576, "MCU"=w573, "Vcell Min (V)"=w577, "appdir"=w548, "errin"=w578, "Température usine (°C)"=21.0, "Tcell Max (°C)"=w575, "Tcell Min (°C)"=w574) -> ("errout"=w572:errorcluster, "datalog"=w580:string, "pass"=w571:bool)  [unwired: 1 out]
            n200 = call <vilib>:"Log_basic.vi"("errin"=w555, "date?"=TRUE, "chaîne"=w580, "in"=w554) -> ("sortie d'erreur"=w552:errorcluster, "refnum en sortie"=w553:refnum<file>)  [unwired: 6 in]
            n201 = call "ZenPlusOP300_refaire.vi"("refaire"=w550, "Pédale"=FALSE, "casOK"=w569, "errin"=w572, "test ok ?"=w571) -> ("errout"=w556:errorcluster, "Next"=w551:T4)  [unwired: 5 in]
            n202 = property on="progression" class="Gliss (strict)"(error in=w556, "Visible"=FALSE, "Value"=u8 0 ("progression")) -> (error out=w549:errorcluster)  [unwired: 1 in, 1 out]
          }
        }
      }
      frame "OCV" {
        (unwired) "Refaire" ("image")
        w612 = OP300ZP_state."Iso" ("Cas OK")
        w602 = enum16{"STR", "DBL", "U32"}."DBL" ("Énum")
        n203 = global read "IS30%.vi" "VG IS30% ?"() -> (w581:bool)
        n204 = call "Mesure OCV"("Enable"=TRUE, "error in (no error)"=w606) -> ("Tension Bat+ Bat-"=w598:dbl, "error out"=w613:errorcluster)  [unwired: 15 in, 1 out]
        n205 = call <vilib>:"FGV_Image.vi"("Énum"=FGV."SET", "IN"="OCV") -> ()  [unwired: 9 in, 1 out]
        n206 = local write "TOP"("Meusure de la tension à vide" ("TOP")) -> ()
        n207 = Select ("Sélectionner")(t="OCV30" ("section"), s=w581, f="OCV70" ("cas faux")) -> (s? t:f=w582:string)
        n208 = call <vilib>:"Application Directory.vi"() -> ("Application Directory"=w601:path)
        n209 = call "Read_Param.vi"("Énum"=w602, "errin"=w613, "pathin"=w601, "section"=w582, "key"="OCVmax") -> ("error out"=w604:errorcluster, "dbl"=w600:dbl)  [unwired: 2 in, 3 out]
        n210 = call "Read_Param.vi"("Énum"=w602, "errin"=w604, "pathin"=w601, "section"=w582, "key"="OCVmin") -> ("error out"=w603:errorcluster, "dbl"=w599:dbl)  [unwired: 2 in, 3 out]
        n211 = In Range and Coerce(upper limit=w600, x=w598, lower limit=w599) -> (In Range?=w591:bool)  [unwired: 1 out]
        n212 = local read "Cluster"() -> (w588:T1)
        n213 = call "ZenPlusOP300_refaire.vi"("refaire"=w585, "casOK"=w612, "errin"=w603, "test ok ?"=w591) -> ("errout"=w592:errorcluster, "Next"=w590:T4)  [unwired: 6 in]
        n214 = Equal?(x=w590, y=w612) -> (x = y?=w611:bool)
        n215 = case shown="Vrai" w611 {
          tunnel: w595 -> [w616 w622]
          tunnel: [w616 w621] -> w594
          tunnel: w597 -> [w615 w620]
          tunnel: [w615 w619] -> w593
          tunnel: w598 -> [_ w618]
          tunnel: ["0" w617] -> w586
          frame False {
          }
          frame True {
            n216 = Number To Decimal String(number=w618) -> (decimal integer string=w617:string)  [unwired: 1 in]
            n217 = Concatenate Strings("OCV;" ("chaîne"), w617) -> (w624:string)
            n218 = call <vilib>:"Log_basic.vi"("errin"=w622, "date?"=TRUE, "chaîne"=w624, "in"=w620) -> ("sortie d'erreur"=w621:errorcluster, "refnum en sortie"=w619:refnum<file>)  [unwired: 6 in]
          }
        }
        n219 = Bundle By Name(cluster=w588, "OCV"=w586) -> (w587:T1)
        n220 = local write "Cluster"(w587) -> ()
      }
    }
    n221 = Wait (ms)(milliseconds to wait=u32 200 ("attente (ms)")) -> ()  [unwired: 1 out]
    n222 = case shown="Faux" w25 {
      selector: w25 -> [_ w32]
      frame False {
      }
      frame True {
        n223 = local write "STOP"(w32) -> ()
      }
    }
  }
  n224 = while {
    shift-right: [w634] -> _
    shift-left: errorcluster {"status"=FALSE, "code"=0, "source"=""} ("error out") -> [w631]
    stop <- w632 stop-if-true
    # "ici tu met l'image à jour si besoin"
    n225 = Wait (ms)(milliseconds to wait=u32 10 ("attente (ms)")) -> ()  [unwired: 1 out]
    n226 = call <vilib>:"FGV_Image.vi"("Énum"=FGV."GET") -> ("OUT"=w627:string)  [unwired: 10 in]
    n227 = Not Equal?(x=w627, y="") -> (x != y?=w628:bool)
    n228 = case shown="Vrai" w628 {
      tunnel: [w636 w641] -> w634
      tunnel: w631 -> [w636 w640]
      tunnel: w627 -> [_ w639]
      frame False {
      }
      frame True {
        n229 = call <vilib>:"Application Directory.vi"() -> ("Application Directory"=w644:path)
        n230 = Path To String(path=w644) -> (string=w645:string)
        n231 = Concatenate Strings(w645, "\\Image\\" ("chaîne"), w639, ".jpg" ("chaîne")) -> (w643:string)
        n232 = call <vilib>:"FGV_Image.vi"("Énum"=FGV."RAZ") -> ()  [unwired: 10 in, 1 out]
        n233 = String To Path(string=w643) -> (path=w642:path)
        n234 = call <vilib>:"Read JPEG File.vi"("error in (no error)"=w640, "path to JPEG file"=w642) -> ("error out"=w641:errorcluster, "image data"=w648:T8)  [unwired: 7 in, 1 out]
        n235 = call <vilib>:"Draw Flattened Pixmap.vi"("image data"=w648) -> ("new picture"=w637:picture)  [unwired: 8 in]
        n236 = local write "DRAW"(w637) -> ()
      }
    }
    n237 = global read "VG_progressBar.vi" "progression"() -> (→"progression":u8)
    n238 = local read "STOP"() -> (w633:bool)
    n239 = Or(x=w634, y=w633) -> (x .or. y?=w632:bool)
  }
  n240 = Merge Errors(w17, w16) -> (→"errout":errorcluster)
  n241 = disable-structure shown="Activé" {
    disable-tunnel: [w649 _] -> _
    frame Disabled {
      n242 = call "Data Dynamiques"() -> ("CMU OK"=w649:bool)  [unwired: 12 in, 7 out]
    }
    frame Enabled {
    }
  }
  "STOP" <- w14
